vi "Plot Load maker V2 - scalewrite wrapper.vi"(5 "X-axis?":bool, 6 "Meta LUT":refnum<data-value>, 7 "Active Scale":i32, 8 "error in (no error)":errorcluster, 9 "Axis config":T1={"Name Label.Text"="", "Style"=0, "Tick Colors:Minor Tick Color"=0, "Tick Colors:Tick Color"=0, "Marker Colors:Text Color"=0, "Grid Colors:Major Color"=0, "Grid Colors:Minor Color"=0, "Mapping Mode"=0, "Flipped"=FALSE, "Name Label.Visible"=FALSE, "Name Label.Text Colors:Text Color"=0, "Scale Fit"=0, "Range:Maximum"=0.0, "Range:Minimum"=0.0, "Offset and Multiplier:Multiplier"=0.0, "Offset and Multiplier:Offset"=0.0, "Name Label.Font:Size"=0, "Marker.Font:Size"=0, "Uniform Marker Spacing?"=TRUE, "Format String"=""}, 10 "spoof":refnum<vi>, 11 "Scale reference":refnum<vi>) -> (0 "error out":errorcluster)   [LabVIEW 2021, in "RocketPlot.lvlib"]
uses:
  RocketPlot.lvlib
  TypeDefs/Plot scale axis properties.ctl
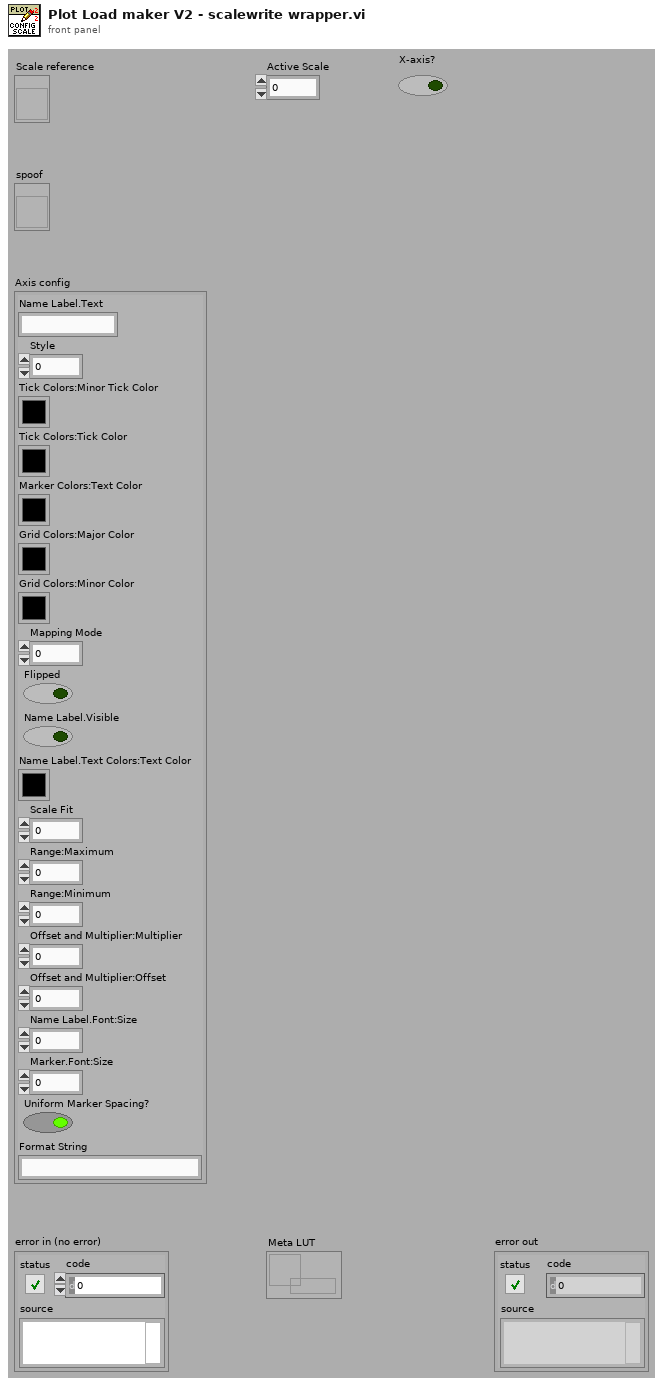
[diagram p1: front panel]
types:
  T1 = typedef "RocketPlot.lvlib/Plot scale axis properties.ctl" = cluster{"Name Label.Text":string, "Style":u8, "Tick Colors:Minor Tick Color":u32, "Tick Colors:Tick Color":u32, "Marker Colors:Text Color":u32, "Grid Colors:Major Color":u32, "Grid Colors:Minor Color":u32, "Mapping Mode":u8, "Flipped":bool, "Name Label.Visible":bool, "Name Label.Text Colors:Text Color":u32, "Scale Fit":u8, "Range:Maximum":dbl, "Range:Minimum":dbl, "Offset and Multiplier:Multiplier":dbl, "Offset and Multiplier:Offset":dbl, "Name Label.Font:Size":u32, "Marker.Font:Size":u32, "Uniform Marker Spacing?":bool, "Format String":string}
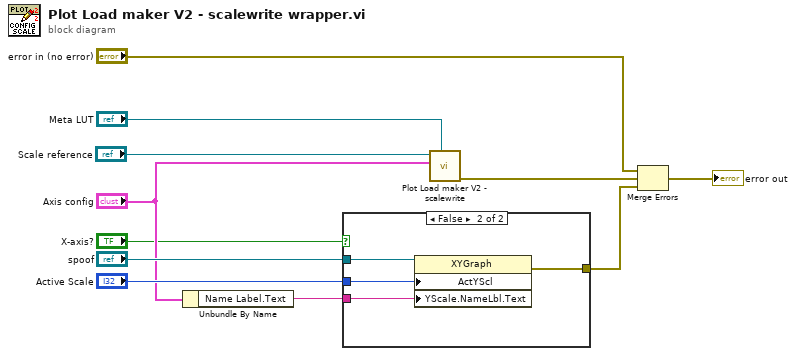
[diagram p0: block diagram]
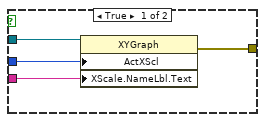
[diagram p2: hidden frame]
diagram:
  n1 = Unbundle By Name("Axis config") -> ("Name Label.Text"=w4:string)
  n2 = case shown="False" "X-axis?" {
    tunnel: [w15 w19] -> w10
    tunnel: "spoof" -> [w14 w18]
    tunnel: "Active Scale" -> [w13 w17]
    tunnel: w4 -> [w12 w16]
    frame True {
      n3 = property class="XYGraph"(reference=w14, "ActXScl"=w13, "XScale.NameLbl.Text"=w12) -> (error out=w15:errorcluster)  [unwired: 1 in, 1 out]
    }
    frame False {
      n4 = property class="XYGraph"(reference=w18, "ActYScl"=w17, "YScale.NameLbl.Text"=w16) -> (error out=w19:errorcluster)  [unwired: 1 in, 1 out]
    }
  }
  n5 = call "Plot Load maker V2 - scalewrite.vi"("Meta LUT"="Meta LUT", "Axis config"="Axis config", "Scale reference"="Scale reference") -> ("error out"=w11:errorcluster)  [unwired: 7 in, 1 out]
  n6 = Merge Errors("error in (no error)", w11, w10) -> (→"error out":errorcluster)
